vi "DIGIT_5122_Init_Session.vi"(7 "Number of Acquisitions":i32, 8 "error in (no error)":errorcluster, 9 "DATA Inputs":T1={"Record Length"=1000000, "Sample Rate"=10000000.0, "Data Type"=0, "Vertical Range"=10.0, "Acquisition Duration"=100000.0} {"Vertical Range" items=["0.2"=0.2, "0.4"=0.4, "1"=1.0, "2"=2.0, "4"=4.0, "10"=10.0]; "Data Type" items=["I16", "DBL"]; "Sample Rate" items=["1 MHz"=1000000.0, "2 MHz"=2000000.0, "5 MHz"=5000000.0, "10 MHz"=10000000.0, "20 MHz"=20000000.0, "25 MHz"=25000000.0, "50 MHz"=50000000.0, "100 MHz"=100000000.0]}, 10 "DIGIT 5122 Inputs":T2={"Sample Rate"=10000.0, "Resource Name"="DIGIT_5122", "Channel Name"="0", "Trigger Source"="VAL_EXTERNAL", "Vertical Range"=10.0, "Trigger Level"=3.0} {"Trigger Level" format="%.2f"; "Vertical Range" format="%.2f"; "Sample Rate" step=65535.0 format="%#_3p"}, 11 "Use Software Trigger":bool) -> (0 "error out":errorcluster, 3 "instrument handle out":refnum<k15>)   [LabVIEW 2017]
doc: "Creates a new IVI instrument driver session. \nOpens a session to the device that you specify in the resource name parameter. \nResets the instrument to a known state if the reset device parameter is set to TRUE.\n\nConfigures the most commonly configured properties of the digitizer vertical subsystem, such as the range, offset, coupling, probe attenuation, and the channel name. \n\nConfigures the common properties of the horizontal subsystem for a single record or multirecord acquisition, such as minimum sample rate and acquisition size. \n\nConfigures common properties for immediate triggering (means the digitizer triggers itself.) or edge triggering (external trigger)."
uses:
  controls/DIGIT_5122_Inputs.ctl
  <instrlib>/niScope/Controls/niScope trigger source.ctl
  controls/DATA_Inputs.ctl
  <instrlib>/niScope/Configure/Trigger/niScope Configure Trigger Edge.vi
  <instrlib>/niScope/Configure/Trigger/niScope Configure Trigger Immediate.vi
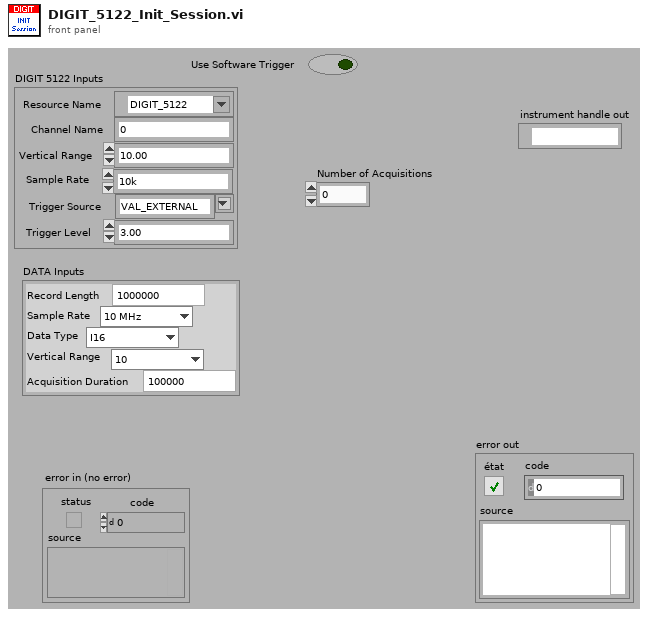
[diagram p1: front panel]
types:
  T1 = typedef "DATA_Inputs.ctl" = cluster{"Record Length":i32, "Sample Rate":dbl, "Data Type":u8, "Vertical Range":dbl, "Acquisition Duration":dbl}
  T2 = typedef "DIGIT_5122_Inputs.ctl" = cluster{"Sample Rate":dbl, "Resource Name":refnum<k15>, "Channel Name":string, "Trigger Source":T3, "Vertical Range":dbl, "Trigger Level":dbl}
  T3 = typedef "niScope trigger source.ctl" = string
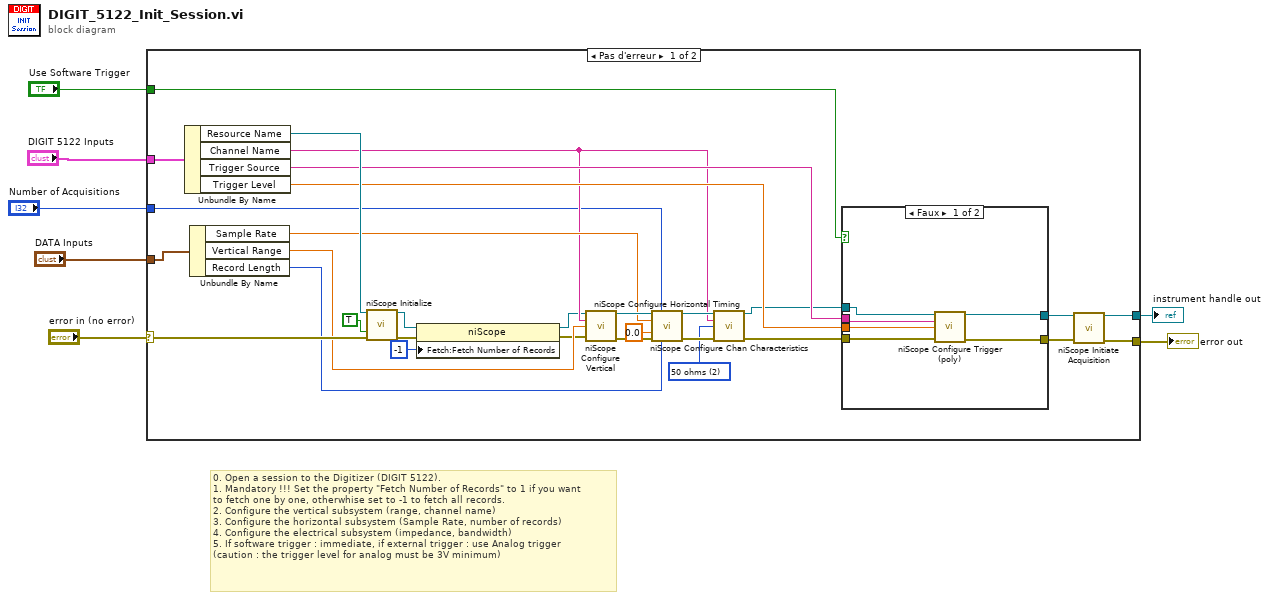
[diagram p0: block diagram]
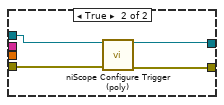
[diagram p2: hidden frame]
diagram:
  # "0. Open a session to the Digitizer (DIGIT 5122).\n1. Mandatory !!! Set the property \"Fetch Number of Records\" to 1 if you want\nto fetch one by one, otherwhise set to -1 to fetch all records.\n2. Configure the vertical subsystem (range, channel name) \n3. Configure the horizontal subsystem (Sample Rate, number of records)\n4. Configure the electrical subsystem (impedance, bandwidth)\n5. If software trigger : immediate, if external trigger : use Analog trigger\n(caution : the trigger level for analog must be 3V minimum)"
  n1 = case shown="Pas d'erreur" "error in (no error)" {
    selector: "error in (no error)" -> [w33 w48]
    tunnel: [w24 w48] -> w7
    tunnel: "Use Software Trigger" -> [w37 _]
    tunnel: [w26 _] -> w3
    tunnel: "DIGIT 5122 Inputs" -> [w36 _]
    tunnel: "DATA Inputs" -> [w21 _]
    tunnel: "Number of Acquisitions" -> [w14 _]
    frame No Error {
      w15 = u32 2 items=["1 mega ohm"=0, "50 ohms"=2] ("input impedance")
      n2 = Unbundle By Name(w36) -> ("Resource Name"=w35:refnum<k15>, "Channel Name"=w16:string, "Trigger Source"=w28:T3, "Trigger Level"=w29:dbl)
      n3 = Unbundle By Name(w21) -> ("Sample Rate"=w23:dbl, "Vertical Range"=w22:dbl, "Record Length"=w30:i32)
      n4 = call <instrlib>:"niScope Initialize.vi"("resource name"=w35, "reset device"=TRUE, "error in"=w33) -> ("instrument handle"=w13:refnum<k15>, "error out"=w11:errorcluster)  [unwired: 11 in]
      n5 = property class="niScope"(reference=w13, error in=w11, "Fetch:Fetch Number of Records"=-1) -> (reference out=w12:refnum<k15>, error out=w10:errorcluster)
      n6 = call <instrlib>:"niScope Configure Vertical.vi"("instrument handle"=w12, "channels"=w16, "vertical range"=w22, "error in"=w10) -> ("instrument handle out"=w32:refnum<k15>, "error out"=w31:errorcluster)  [unwired: 10 in]
      n7 = call <instrlib>:"niScope Configure Horizontal Timing.vi"("instrument handle"=w32, "number of records"=w14, "min sample rate"=w23, "reference position"=0.0, "error in"=w31, "min record length"=w30) -> ("instrument handle out"=w20:refnum<k15>, "error out"=w19:errorcluster)  [unwired: 8 in]
      n8 = call <instrlib>:"niScope Configure Chan Characteristics.vi"("instrument handle"=w20, "channels"=w16, "input impedance"=w15, "error in"=w19) -> ("instrument handle out"=w17:refnum<k15>, "error out"=w18:errorcluster)  [unwired: 10 in]
      n9 = case shown="Faux" w37 {
        tunnel: [w41 w47] -> w27
        tunnel: [w40 w46] -> w25
        tunnel: w29 -> [w43 _]
        tunnel: w28 -> [w42 _]
        tunnel: w17 -> [w39 w45]
        tunnel: w18 -> [w38 w44]
        frame False {
          n10 = call-poly <instrlib>:"niScope Configure Trigger (poly).vi"("instrument handle"=w39, "trigger source"=w42, "trigger level"=w43, "error in"=w38) -> ("instrument handle out"=w41:refnum<k15>, "error out"=w40:errorcluster)  [unwired: 10 in]
        }
        frame True {
          n11 = call-poly <instrlib>:"niScope Configure Trigger (poly).vi"("instrument handle"=w45, "error in"=w44) -> ("instrument handle out"=w47:refnum<k15>, "error out"=w46:errorcluster)  [unwired: 12 in]
        }
      }
      n12 = call <instrlib>:"niScope Initiate Acquisition.vi"("instrument handle"=w27, "error in"=w25) -> ("instrument handle out"=w26:refnum<k15>, "error out"=w24:errorcluster)  [unwired: 12 in]
    }
    frame Error {
    }
  }
  "error out" <- w7
  "instrument handle out" <- w3
